vi "populateTelemetryHardpointStatus.vi"(8 "error in (no error)":errorcluster, 11 "Model in":refnum<class "Model.lvclass">) -> (0 "error out":errorcluster, 3 "Model out":refnum<class "Model.lvclass">)   [LabVIEW 2016, in "Model.lvclass"]
uses:
  Model.lvclass
  Model.lvclass/Model.ctl
  ILCCommunications/ILCCommunications.lvclass/ILCCommunications.ctl
  Publisher/Publisher.lvclass/Publisher.ctl
  Common_RT_ILC/ILC/ILC.lvclass/ILC.ctl
  Common_RT_HPILC/HPILC/HPILC.lvclass
  D:/Code/ts_M1M3Support/Common_RT_ILC/ILC/ILC.lvclass
  ILCCommunications/ILCCommunications.lvclass
  Publisher/Publisher.lvclass
  Common_RT_ILC/ILC/ILC.lvclass
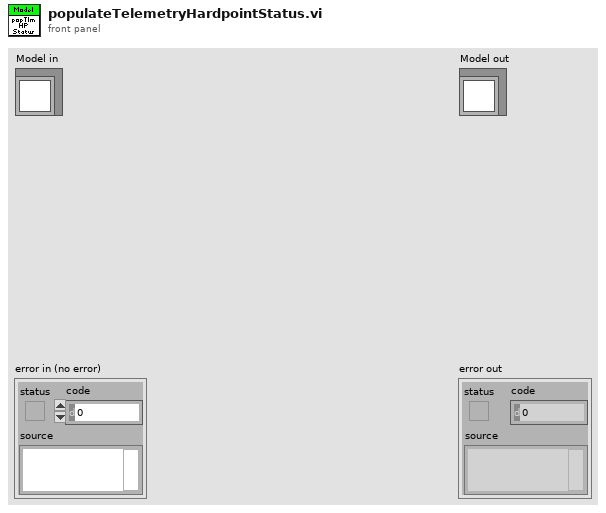
[diagram p1: front panel]
types:
  T1 = typedef "RTILC.lvlib/ILCData.ctl" = cluster{"Constants":T2, "Command":T3, "Telemetry":T5, "Responses":T6, "Timestamps":T8, "Timings":T9}
  T2 = typedef "RTILC.lvlib/ILCConstants.ctl" = cluster{"Subnet":u8, "Address":u8}
  T3 = typedef "RTILC.lvlib/ILCCommand.ctl" = cluster{"Mode":u16, "TemporaryAddress":u8, "ADCScanRate":T4, "ADCChannel":u8, "ADCOffset":sgl, "ADCSensitivity":sgl}
  T4 = typedef "RTILC.lvlib/ILCScanRates.ctl" = u8
  T5 = typedef "RTILC.lvlib/ILCTelemetry.ctl" = cluster{"UniqueID":u64, "FirmwareType":u8, "NetworkNodeType":u8, "ILCOption":u8, "NetworkNodeOption":u8, "MajorRevision":u8, "MinorRevision":u8, "FirmwareName":string, "Mode":u16, "MajorFault":bool, "MinorFault":bool, "FaultOverride":bool, "MainCalibrationError":bool, "BackupCalibrationError":bool, "UniqueIDCRCMismatch":bool, "AppTypeNodeTypeMismatch":bool, "AppMissing":bool, "AppCRCMismatch":bool, "TEDSNotFound":bool, "TEDS1Mismatch":bool, "TEDS2Mismatch":bool, "WatchdogResetDetected":bool, "BrownoutDetected":bool, "EventTrapResetDetected":bool, "MotorPowerFault":bool, "SSRPowerFault":bool, "AuxPowerFault":bool, "SMCPowerFault":bool, "TemporaryAddress":u8, "ADCScanRate":T4, "MainADCCalibrationK":sgl[], "MainSensorOffset":sgl[], "MainSensorSensitivity":sgl[], "BackupADCCalibrationK":sgl[], "BackupSensorOffset":sgl[], "BackupSensorSensitivity":sgl[]}
  T6 = typedef "RTILC.lvlib/ILCResponses.ctl" = cluster{"ReportServerID":T7, "ReportServerStatus":T7, "Mode":T7, "TemporaryAddress":T7, "Reset":T7, "ADCScanRate":T7, "ADCOffsetSensitivity":T7, "ReportCalibrationData":T7}
  T7 = typedef "RTModbus.lvlib/ExceptionCodes.ctl" = u16
  T8 = typedef "RTILC.lvlib/ILCTimestamps.ctl" = cluster{"ReportServerID":dbl, "ReportServerStatus":dbl, "Mode":dbl, "TemporaryAddress":dbl, "Reset":dbl, "ADCScanRate":dbl, "ADCOffsetSensitivity":dbl, "ReportCalibrationData":dbl}
  T9 = typedef "RTILC.lvlib/ILCTimings.ctl" = cluster{"ReportServerID":u32, "ReportServerStatus":u32, "Mode":u32, "TemporaryAddress":u32, "Reset":u32, "ADCScanRate":u32, "ADCOffsetSensitivity":u32, "ReportCalibrationData":u32}
  T10 = typedef "M1M3SupportTopics.lvlib/Timestamp.ctl" = dbl
  T11 = typedef "M1M3SupportTopics.lvlib/TelemetryHardpointStatus.ctl" = cluster{"Timestamp":T10, "Mode":u8[], "MajorFault":bool[], "MinorFault":bool[], "FaultOverridden":bool[], "WatchdogReset":bool[], "BrownoutDetected":bool[], "EventTrapReset":bool[], "MotorPowerFault":bool[], "SSRPowerFault":bool[], "AUXPowerFault":bool[], "SMCPowerFault":bool[]}
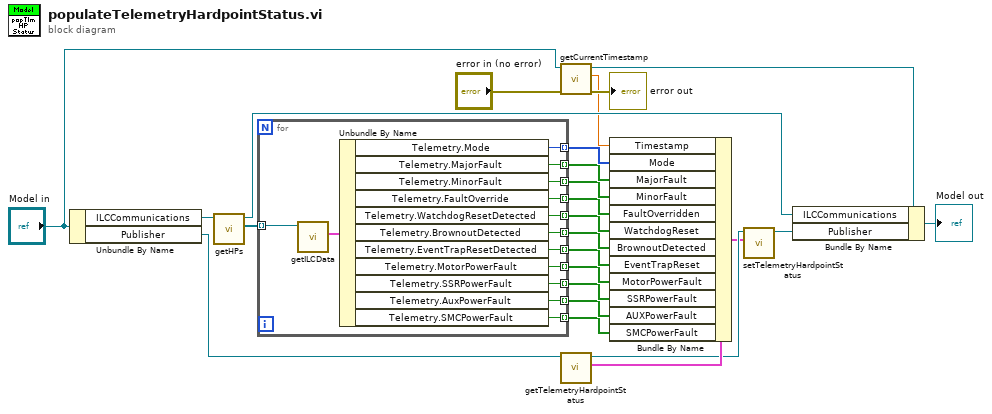
[diagram p0: block diagram]
diagram:
  n1 = Unbundle By Name("Model in") -> ("ILCCommunications"=w24:refnum<class "ILCCommunications.lvclass">, "Publisher"=w23:refnum<class "Publisher.lvclass">)
  n2 = call "getHPs.vi"("ILCCommunications in"=w24) -> ("HPs"=w20:refnum<class "HPILC.lvclass">[], "ILCCommunications out"=w18:refnum<class "ILCCommunications.lvclass">)  [unwired: 9 in]
  n3 = for {
    tunnel: w20 -> [w38] mode=indexing
    tunnel: [w36] -> w12 mode=indexing
    tunnel: [w35] -> w11 mode=indexing
    tunnel: [w34] -> w10 mode=indexing
    tunnel: [w33] -> w9 mode=indexing
    tunnel: [w32] -> w8 mode=indexing
    tunnel: [w31] -> w7 mode=indexing
    tunnel: [w30] -> w6 mode=indexing
    tunnel: [w29] -> w5 mode=indexing
    tunnel: [w28] -> w4 mode=indexing
    tunnel: [w27] -> w3 mode=indexing
    tunnel: [w26] -> w2 mode=indexing
    n4 = call "getILCData.vi"("ILC in"=w38) -> ("ILCData"=w37:T1)  [unwired: 9 in, 1 out]
    n5 = Unbundle By Name(w37) -> ("Telemetry.Mode"=w36:u16, "Telemetry.MajorFault"=w35:bool, "Telemetry.MinorFault"=w34:bool, "Telemetry.FaultOverride"=w33:bool, "Telemetry.WatchdogResetDetected"=w32:bool, "Telemetry.BrownoutDetected"=w31:bool, "Telemetry.EventTrapResetDetected"=w30:bool, "Telemetry.MotorPowerFault"=w29:bool, "Telemetry.SSRPowerFault"=w28:bool, "Telemetry.AuxPowerFault"=w27:bool, "Telemetry.SMCPowerFault"=w26:bool)
  }
  n6 = call "getCurrentTimestamp.vi"("error in (no error)"="error in (no error)", "Model in"="Model in") -> ("error out"=→"error out":errorcluster, "Timestamp"=w1:T10, "Model out"=w16:refnum<class "Model.lvclass">)  [unwired: 7 in]
  n7 = call "getTelemetryHardpointStatus.vi"("Publisher in"=w23) -> ("TelemetryHardpointStatus"=w22:T11, "Publisher out"=w21:refnum<class "Publisher.lvclass">)  [unwired: 9 in]
  n8 = Bundle By Name(cluster=w22, "Timestamp"=w1, "Mode"=w12, "MajorFault"=w11, "MinorFault"=w10, "FaultOverridden"=w9, "WatchdogReset"=w8, "BrownoutDetected"=w7, "EventTrapReset"=w6, "MotorPowerFault"=w5, "SSRPowerFault"=w4, "AUXPowerFault"=w3, "SMCPowerFault"=w2) -> (w13:T11)
  n9 = call "setTelemetryHardpointStatus.vi"("TelemetryHardpointStatus"=w13, "Publisher in"=w21) -> ("Publisher out"=w19:refnum<class "Publisher.lvclass">)  [unwired: 9 in]
  n10 = Bundle By Name(cluster=w16, "ILCCommunications"=w18, "Publisher"=w19) -> (→"Model out":refnum<class "Model.lvclass">)
